vi "configuration object to database element.vi"(8 "error in":errorcluster, 11 "configuration in":refnum<class "TBM configuration.lvclass">) -> (0 "error out":errorcluster, 3 "database":T1)   [LabVIEW 2013, in "PLConfigurationSerializer.lvlib"]
uses:
  PLConfigurationSerializer.lvlib
  configuration database.ctl
  <vilib>/NI/Tag Bus Module Framework/root configuration/TBM configuration.lvclass
  <vilib>/NI/CEF/CEF_TreeControl/serializable configuration/NISE_CEF_serializable configuration.lvclass
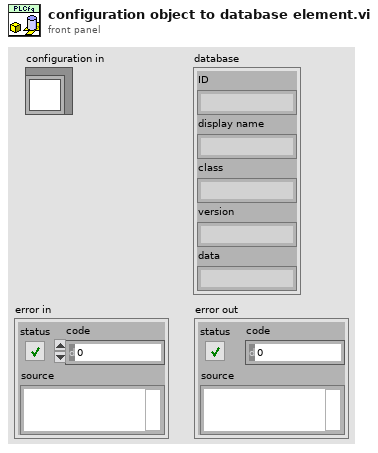
[diagram p1: front panel]
types:
  T1 = typedef "PLConfigurationSerializer.lvlib/configuration database.ctl" = cluster{"ID":string, "display name":string, "class":string, "version":string, "data":string}
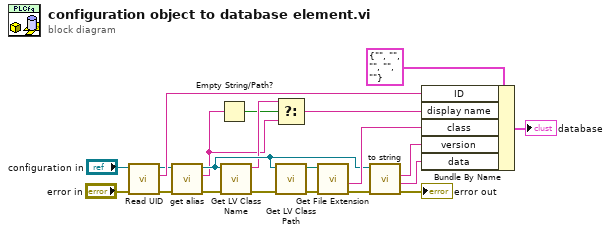
[diagram p0: block diagram]
diagram:
  n1 = call <vilib>:"Read UID.vi"("error in"="error in", "configuration in"="configuration in") -> ("error out"=w6:errorcluster, "instance id"=w10:string, "configuration out"=w7:refnum<class "TBM configuration.lvclass">)  [unwired: 7 in]
  n2 = call <vilib>:"get alias.vi"("error in"=w6, "configuration in"=w7) -> ("error out"=w5:errorcluster, "alias"=w1:string, "configuration out"=w4:refnum<class "TBM configuration.lvclass">)  [unwired: 7 in]
  n3 = Empty String/Path?(string/path=w1) -> (empty?=w2:bool)
  n4 = call <vilib>:"Get LV Class Name.vi"("error in (no error)"=w5, "object"=w4) -> ("error out"=w9:errorcluster, "class name"=w3:string)  [unwired: 8 in]
  n5 = Select(t=w3, s=w2, f=w1) -> (s? t:f=w8:string)
  n6 = call <vilib>:"Get LV Class Path.vi"("error in (no error)"=w9, "object"=w4) -> ("error out"=w16:errorcluster, "class path"=w14:path)  [unwired: 8 in]
  n7 = call <vilib>:"Get File Extension.vi"("error in (no error)"=w16, "file"=w14) -> ("error out"=w15:errorcluster, "filename without extension"=w13:string)  [unwired: 6 in, 2 out]
  n8 = call-dynamic "to string.vi"("error in"=w15, "configuration in"=w4) -> ("error out"=→"error out":errorcluster, "data"=w18:string, "version"=w17:string)  [unwired: 6 in, 1 out]
  n9 = Bundle By Name(cluster=T1 {"ID"="", "display name"="", "class"="", "version"="", "data"=""} ("database"), "ID"=w10, "display name"=w8, "class"=w13, "version"=w17, "data"=w18) -> (→"database":T1)
